vi "Set G08 Clock Parameters.vi"(4 "Trigger Multiplier":u32=4, 6 "Trigger Divider":u32=1, 7 "DG Number":i32, 8 "error in (no error)":errorcluster, 9 "Clock Source":u32(ring)=3 items=["Internal Oscillator"=1, "External Trigger"=2, "Trigger & Oscillator"=3, "Master Slave Bus"=4], 10 "Ocillator Divider":u32=2, 11 "Clock Enable":bool=TRUE) -> (0 "error out":errorcluster)   [LabVIEW 2009, in "POLARIS BME DG.lvlib"]
doc: "long Set_ClockParameters(BOOL ClockEnable, unsigned long DivideBy, unsigned long ClockSource, long DG_Number);"
uses:
  POLARIS BME DG.lvlib
  BME DLL/DelayGenerator.dll
panel:
  # "NOTICE -- YOU MUST LEAVE THIS NOTICE IN PLACE.  PER THE TERMS OF THE LICENSE BELOW, YOU MAY SUBLICENSE THIS SOFTWARE \nIN ANY WAY THAT DOES NOT CONFLICT WITH THIS LICENSE.\n\n### BSD License (http://www.opensource.org/licenses/bsd-license.php) Begin ###\n \nCopyright (c) 2011, Applied Energetics, http://www.appliedenergetics.com,\n                               Richard Schwerdtfeger, <rschwerdtfeger@appliedenergetics.com>\n\nAll rights reserved.\n\nRedistribution and use in source and binary forms, with or without modification, are permitted provided that the \nfollowing conditions are met:\n\n    * Redistributions of source code must retain the above copyright notice, this list of conditions and the following disclaimer.\n    * Redistributions in binary form must reproduce the above copyright notice, this list of conditions and the following disclaimer \n       in the documentation and/or other materials provided with the distribution.\n    * Neither the name of Richard Schwerdtfeger, Applied Energetics, Inc., nor the names of its contributors may be used to \n       endorse or promote products derived from this software without specific prior written permission.\n\nTHIS SOFTWARE IS PROVIDED BY THE COPYRIGHT HOLDERS AND CONTRIBUTORS \"AS IS\" AND ANY EXPRESS OR IMPLIED WARRANTIES, \nINCLUDING, BUT NOT LIMITED TO, THE IMPLIED WARRANTIES OF MERCHANTABILITY AND FITNESS FOR A PARTICULAR PURPOSE ARE \nDISCLAIMED. IN NO EVENT SHALL THE COPYRIGHT OWNER OR CONTRIBUTORS BE LIABLE FOR ANY DIRECT, INDIRECT, INCIDENTAL,\n SPECIAL, EXEMPLARY, OR CONSEQUENTIAL DAMAGES (INCLUDING, BUT NOT LIMITED TO, PROCUREMENT OF SUBSTITUTE GOODS OR \nSERVICES; LOSS OF USE, DATA, OR PROFITS; OR BUSINESS INTERRUPTION) HOWEVER CAUSED AND ON ANY THEORY OF LIABILITY, \nWHETHER IN CONTRACT, STRICT LIABILITY, OR TORT (INCLUDING NEGLIGENCE OR OTHERWISE) ARISING IN ANY WAY OUT OF THE USE \nOF THIS SOFTWARE, EVEN IF ADVISED OF THE POSSIBILITY OF SUCH DAMAGE.\n\n### BSD License End ###"
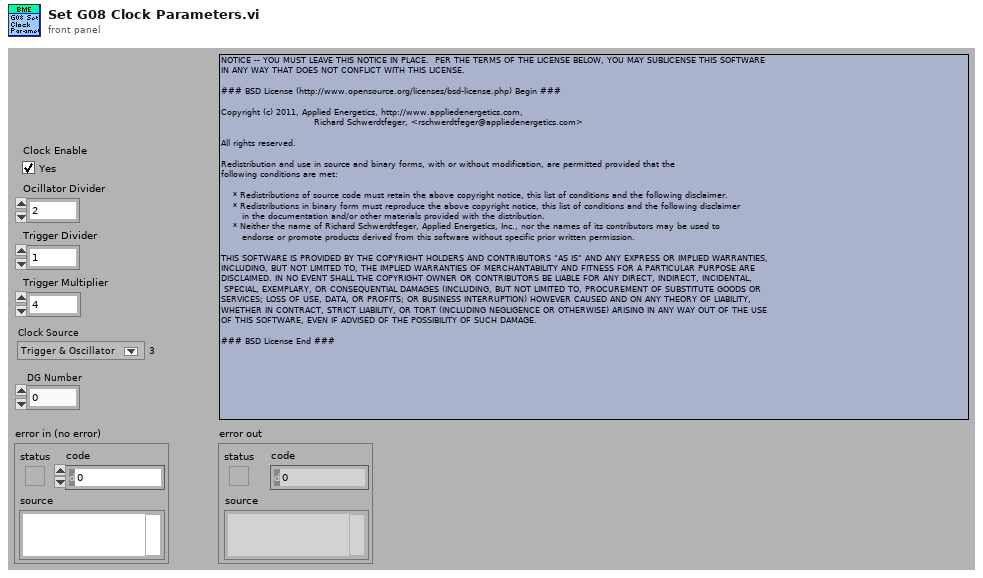
[diagram p1: front panel]
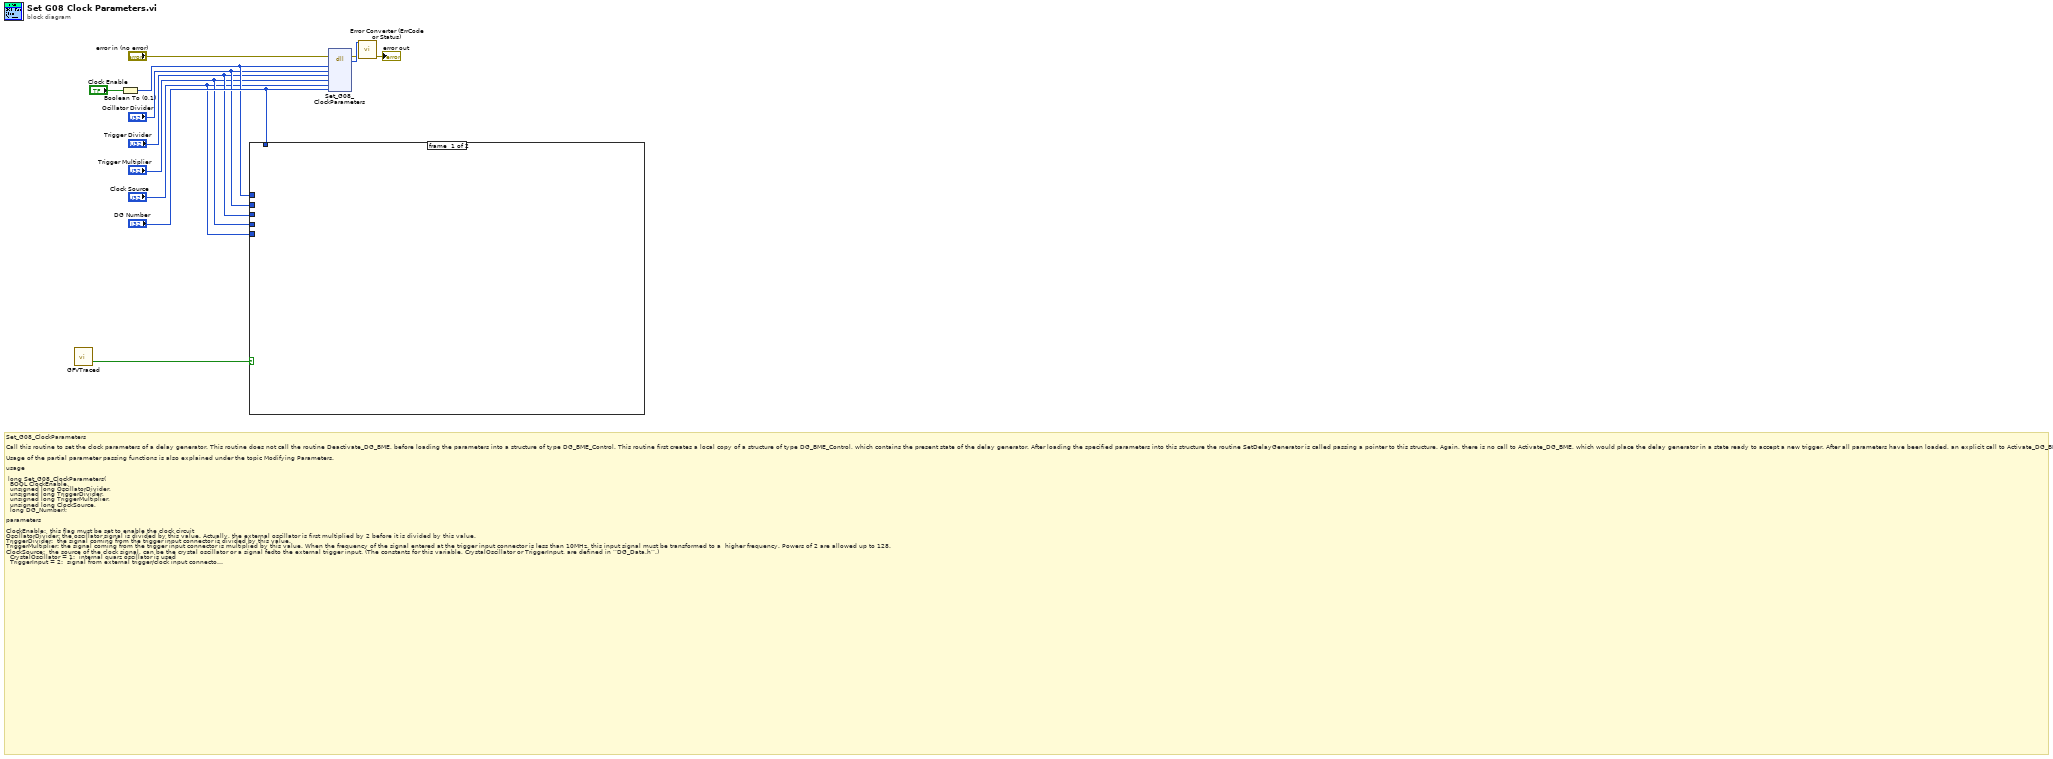
[diagram p0: block diagram]
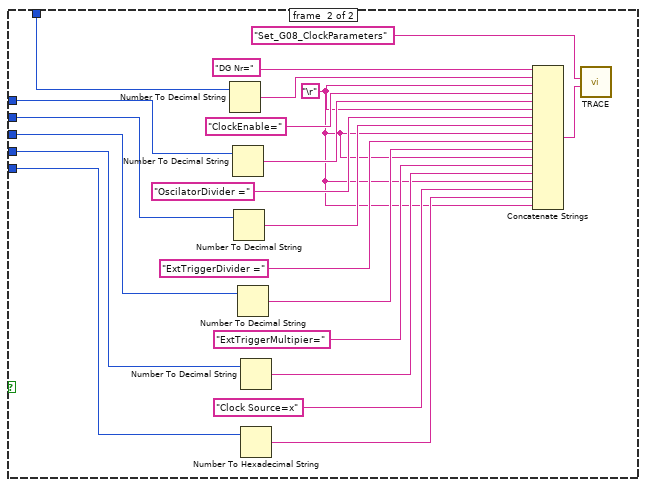
[diagram p2: hidden frame]
diagram:
  # "Set_G08_ClockParameters\n\nCall this routine to set the clock parameters of a delay generator. This routine does not call the routine Deactivate_DG_BME, before loading the parameters into a structure of type DG_BME_Control. This routine first creates a local copy of a structure of type DG_BME_Control, which contains the present state of the delay generator. After loading the specified parameters into this structure the routine SetDelayGenerator is called passing a pointer to this structure. Again, there is no call to Activate_DG_BME, which would place the delay generator in a state ready to accept a new trigger. After all parameters have been loaded, an explicit call to Activate_DG_BME is necessary.\n\nUsage of the partial parameter passing functions is also explained under the topic Modifying Parameters.\n\nusage\n\n long Set_G08_ClockParameters(\n\t\tBOOL ClockEnable, \n\t\tunsigned long OscillatorDivider, \n\t\tunsigned long TriggerDivider, \n\t\tunsigned long TriggerMultiplier, \n\t\tunsigned long ClockSource,\n\t\tlong DG_Number);\n\nparameters\n\nClockEnable:\t\tthis flag must be set to enable the clock circuit\nOscillatorDivider:\tthe oscillator signal is divided by this value. Actually, the external oscillator is first multiplied by 2 before it is divided by this value.\nTriggerDivider:\t\tthe signal coming from the trigger input connector is divided by this value. \nTriggerMultiplier:\tthe signal coming from the trigger input connector is multiplied by this value. When the frequency of the signal entered at the trigger input connector is less than 10MHz, this input signal must be transformed to a  higher frequency. Powers of 2 are allowed up to 128.\nClockSource:\t\tthe source of the clock signal, can be the crystal oscillator or a signal fedto the external trigger input. (The constants for this variable, CrystalOscillator or TriggerInput, are defined in ‘’DG_Data.h’’.)\n  CrystalOscillator = 1:\t\tinternal quarz oscillator is used\n  TriggerInput = 2:\t\tsignal from external trigger/clock input connector is used\n  TriggerAndOscillator = 3: \tlike TriggerInput, but if this signal fails, the signal from the internal quarz oscillator will be used.\n\nMasterSlaveBus = 4: \t\tthe clock signal transmitted from the master card is used.\nDG_Number:\t\tThe number of the delay generator as assigned by the\n\nInitialize_DG_BME routine\n\nreturn value\n\n\t0:  success\n\t2:  DG_Number is out of range\n\t7:  parameter ‘ClockSource’ has been passed with illegal value. (See DG_Data.h)"
  n1 = call "GFVTraced.vi"() -> ("traced?"=w7:bool)  [unwired: 2 in]
  n2 = Boolean To (0,1)(Boolean="Clock Enable") -> (0, 1=w5:i16)
  n3 = case shown="True" w7 {
    tunnel: "DG Number" -> [_ w18]
    tunnel: w5 -> [_ w17]
    tunnel: "Ocillator Divider" -> [_ w16]
    tunnel: "Trigger Divider" -> [_ w15]
    tunnel: "Trigger Multiplier" -> [_ w14]
    tunnel: "Clock Source" -> [_ w13]
    frame #0 {
    }
    frame #1 {
      w19 = "\r"
      n4 = Number To Decimal String(number=w18) -> (decimal integer string=w30:string)  [unwired: 1 in]
      n5 = Number To Decimal String(number=w17) -> (decimal integer string=w28:string)  [unwired: 1 in]
      n6 = Number To Decimal String(number=w16) -> (decimal integer string=w26:string)  [unwired: 1 in]
      n7 = Number To Decimal String(number=w15) -> (decimal integer string=w24:string)  [unwired: 1 in]
      n8 = Number To Decimal String(number=w14) -> (decimal integer string=w22:string)  [unwired: 1 in]
      n9 = Number To Hexadecimal String(2:w13) -> (0:w20:string)  [unwired: 1 in]
      n10 = Concatenate Strings("DG Nr=", w30, w19, "ClockEnable=", w28, w19, "OscilatorDivider =", w26, w19, "ExtTriggerDivider =", w24, w19, "ExtTriggerMultipier=", w22, w19, "Clock Source=x", w20, w19) -> (w31:string)
      n11 = call "TRACE.vi"("Parameter String"=w31, "Function"="Set_G08_ClockParameters") -> ()  [unwired: 10 in]
    }
  }
  n12 = dll-call lib="D:/CS Framework/LVSCC/LV2009/GPL/Projects/cs-framework/CSClass/CSPOLARIS/POLARIS BME DG/BME DLL/DelayGenerator.dll" fn="Set_G08_ClockParameters"(error in="error in (no error)", "ClockEnable"=w5, "OscillatorDivider"="Ocillator Divider", "TriggerDivider"="Trigger Divider", "TriggerMultiplier"="Trigger Multiplier", "ClockSource"="Clock Source", "DG_Number"="DG Number") -> (error out=w9:errorcluster, "return type"=w12:i32)  [unwired: 8 in, 1 out]
  n13 = call "Error Converter (ErrCode or Status).vi"("error in (no error)"=w9, "error code"=w12) -> ("error out"=→"error out":errorcluster)  [unwired: 9 out]
